vi "12_4_1_1 - Smoothing.vi"() -> ()   [LabVIEW 2013]
uses:
  <vilib>/Analysis/2dsp.llb/2D Convolution (DBL).vi
  <vilib>/Analysis/NI_AALPro.lvlib
panel:
  out "smoothing (b)":dbl[][](graph)
  out "Source Image (a)":u8[][](graph)
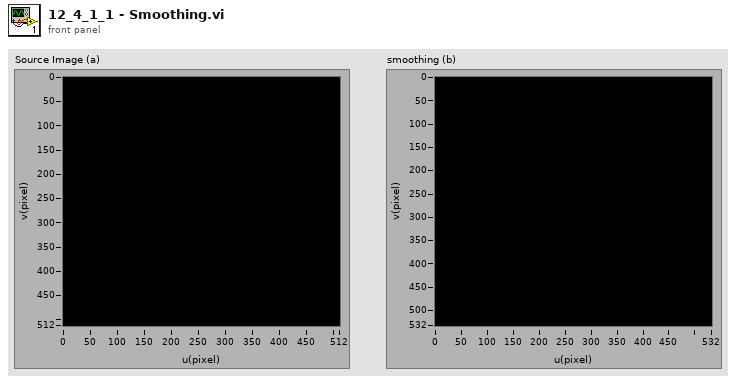
[diagram p1: front panel]
types:
  T1 = typedef "imagedata.ctl" = cluster{"image type":i32, "image depth":i32, "image":u8[], "mask":u8[], "colors":u32[], "Rectangle":cluster{"left":i16, "top":i16, "right":i16, "bottom":i16}}
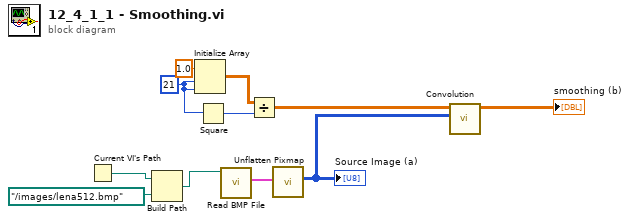
[diagram p0: block diagram]
diagram:
  w3 = 21 ("matrix size")
  n1 = Current VI's Path() -> (path=w10:path)
  n2 = Build Path(base path=w10, name or relative path=path "../images/lena512.bmp") -> (appended path=w11:path)
  n3 = Initialize Array(1.0 ("element"), w3, w3) -> (w5:dbl[][])
  n4 = Square(x=w3) -> (x^2=w6:i32)
  n5 = call <vilib>:"Read BMP File.vi"("path to BMP file"=w11) -> ("image data"=w8:T1)  [unwired: 8 in, 2 out]
  n6 = Divide(x=w5, y=w6) -> (x/y=w1:dbl[][])
  n7 = call <vilib>:"Unflatten Pixmap.vi"("image data"=w8) -> ("8-bit pixmap"=w4:u8[][])  [unwired: 4 in, 6 out]
  "Source Image (a)" <- w4
  n8 = call-poly <vilib>:"Convolution.vi"("Y"=w4, "X"=w1) -> ("X * Y"=→"smoothing (b)":dbl[][])  [unwired: 8 in, 1 out]
